vi "Set As Dialog.vi"(5 "error in (no error)":errorcluster, 6 "Modal? (T)":bool=TRUE, 7 "Allow menu? (F)":bool, 8 "Only in RTE (T)":bool=TRUE) -> (0 "error out":errorcluster)   [LabVIEW 2013]
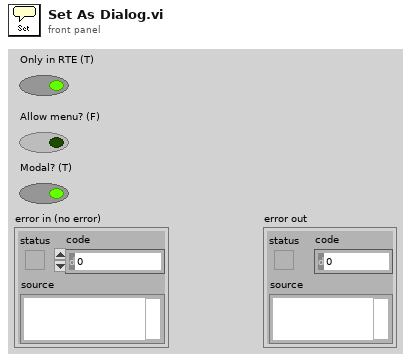
[diagram p1: front panel]
types:
  T1 = enum32{"Invalid", "Standard", "Closed", "Hidden", "Minimized", "Maximized"}
  T2 = enum16{"Always On", "Always Off", "Off While Running"}
  T3 = enum32{"Invalid", "Default", "Floating", "Floating/Auto-Hide", "Modal"}
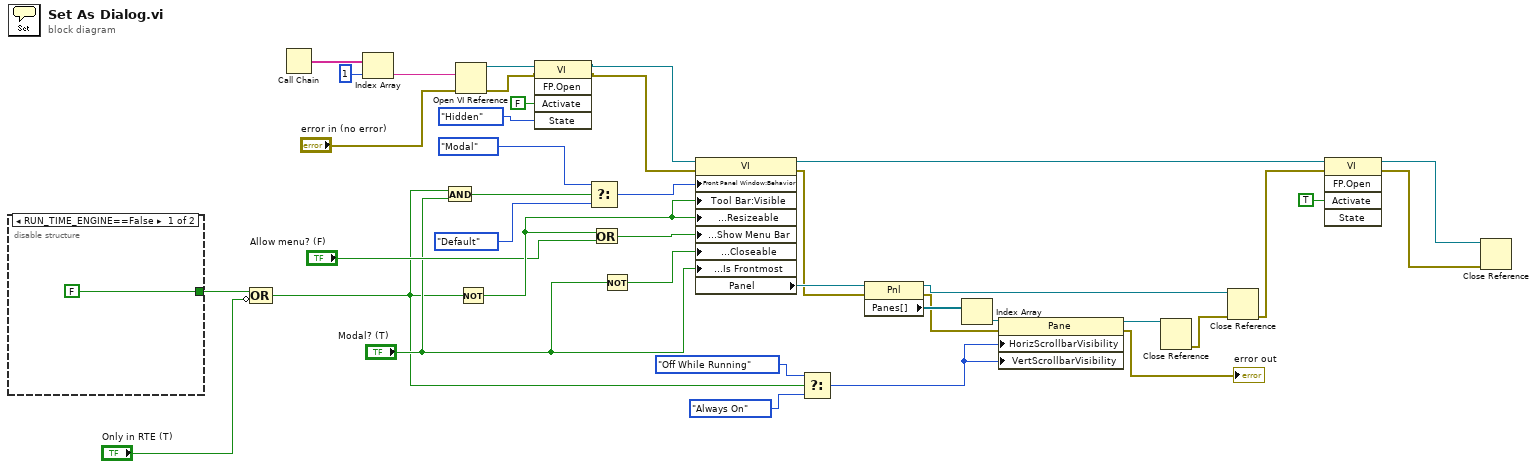
[diagram p0: block diagram]
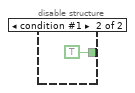
[diagram p2: hidden frame]
diagram:
  n1 = disable-structure shown="RUN_TIME_ENGINE==False" {
    disable-tunnel: [FALSE ("exe-file?") TRUE ("exe-file?")] -> w13
    frame condition #0 (active) {
    }
    frame condition #1 {
    }
  }
  n2 = Compound Arithmetic op=OR(w13, invert "Only in RTE (T)") -> (w12:bool)
  n3 = Call Chain() -> (call chain=w39:string[])
  n4 = Index Array(array=w39, index=1) -> (element=w37:string)
  n5 = And(x=w12, y="Modal? (T)") -> (x .and. y?=w28:bool)
  n6 = Open VI Reference(vi path=w37, error in (no error)="error in (no error)") -> (vi reference=w6:refnum<vi>, error out=w3:errorcluster)  [unwired: 4 out]
  n7 = Not(x=w12) -> (.not. x?=w32:bool)
  n8 = invoke class="VI" method="FP.Open"(reference=w6, error in=w3, "Activate"=FALSE ("Activate?"), "State"=T1."Hidden" ("Front Panel Window:State")) -> (reference out=w5:refnum<vi>, error out=w4:errorcluster)  [unwired: 1 in, 3 out]
  n9 = Select(t=T3."Modal" ("Front Panel Window:Behavior"), s=w28, f=T3."Default" ("Front Panel Window:Behavior")) -> (s? t:f=w34:T3)
  n10 = Or(x=w32, y="Allow menu? (F)") -> (x .or. y?=w30:bool)
  n11 = Not(x="Modal? (T)") -> (.not. x?=w33:bool)
  n12 = property class="VI"(reference=w5, error in=w4, "Front Panel Window:Behavior"=w34, "Tool Bar:Visible"=w32, "Front Panel Window:Resizeable"=w32, "Front Panel Window:Show Menu Bar"=w30, "Front Panel Window:Closeable"=w33, "Front Panel Window:Is Frontmost"="Modal? (T)") -> (reference out=w10:refnum<vi>, error out=w18:errorcluster, "Panel"=w27:refnum<vi>)
  n13 = Select(t=T2."Off While Running" ("Vertical Scrollbar Visibility"), s=w12, f=T2."Always On" ("Vertical Scrollbar Visibility")) -> (s? t:f=w22:T2)
  n14 = property class="Pnl"(reference=w27, error in=w18) -> (reference out=w19:refnum<vi>, error out=w17:errorcluster, "Panes[]"=w26:refnum<vi>[])
  n15 = Index Array(array=w26) -> (element=w25:refnum<vi>)  [unwired: 1 in]
  n16 = property class="Pane"(reference=w25, error in=w17, "HorizScrollbarVisibility"=w22, "VertScrollbarVisibility"=w22) -> (reference out=w21:refnum<vi>, error out=→"error out":errorcluster)
  n17 = Close Reference(reference=w21) -> (error out=w20:errorcluster)  [unwired: 1 in]
  n18 = Close Reference(reference=w19, error in (no error)=w20) -> (error out=w9:errorcluster)
  n19 = invoke class="VI" method="FP.Open"(reference=w10, error in=w9, "Activate"=TRUE ("Activate?")) -> (reference out=w8:refnum<vi>, error out=w7:errorcluster)  [unwired: 2 in, 3 out]
  n20 = Close Reference(reference=w8, error in (no error)=w7) -> ()  [unwired: 1 out]
